vi "MH_CalcDeltaT_EB.vi"(0 "WinDelta":i32, 1 "TrueTime":u64, 2 "WIndowW":i32, 3 "Buffsize":i32, 4 "DBuffSize":i32=10, 5 "Data In":u64[](array[numeric]), 7 "DeltasBuffer":i32[](array[numeric]), 9 "Deltaindex":i32, 11 "error In":errorcluster, 12 "WinIndex":i32, 13 "queue out":refnum<queue>) -> (6 "DeltasBufferOut":i32[](array[numeric]), 8 "DeltaIndexOut":i32, 10 "NewDelta":bool, 14 "WinIndexOut":i32, 15 "Error Out":errorcluster caption="error Out")   [LabVIEW 2019]
uses:
  <userlib>/MultiHarp150/T2Lib/MH_T2DeltaQMessage.ctl
panel:
  # "here"
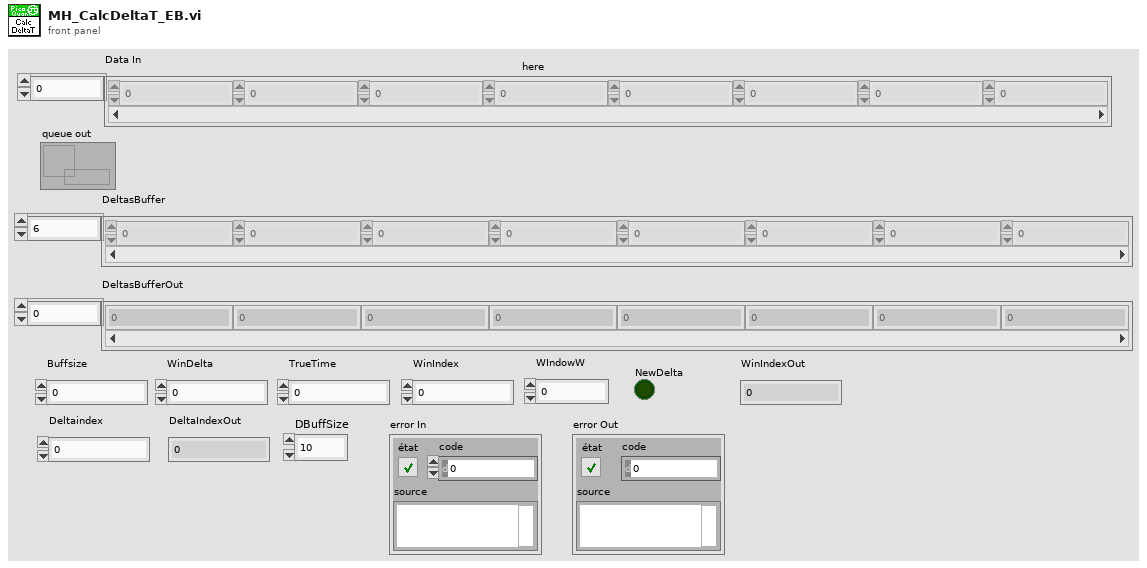
[diagram p1: front panel]
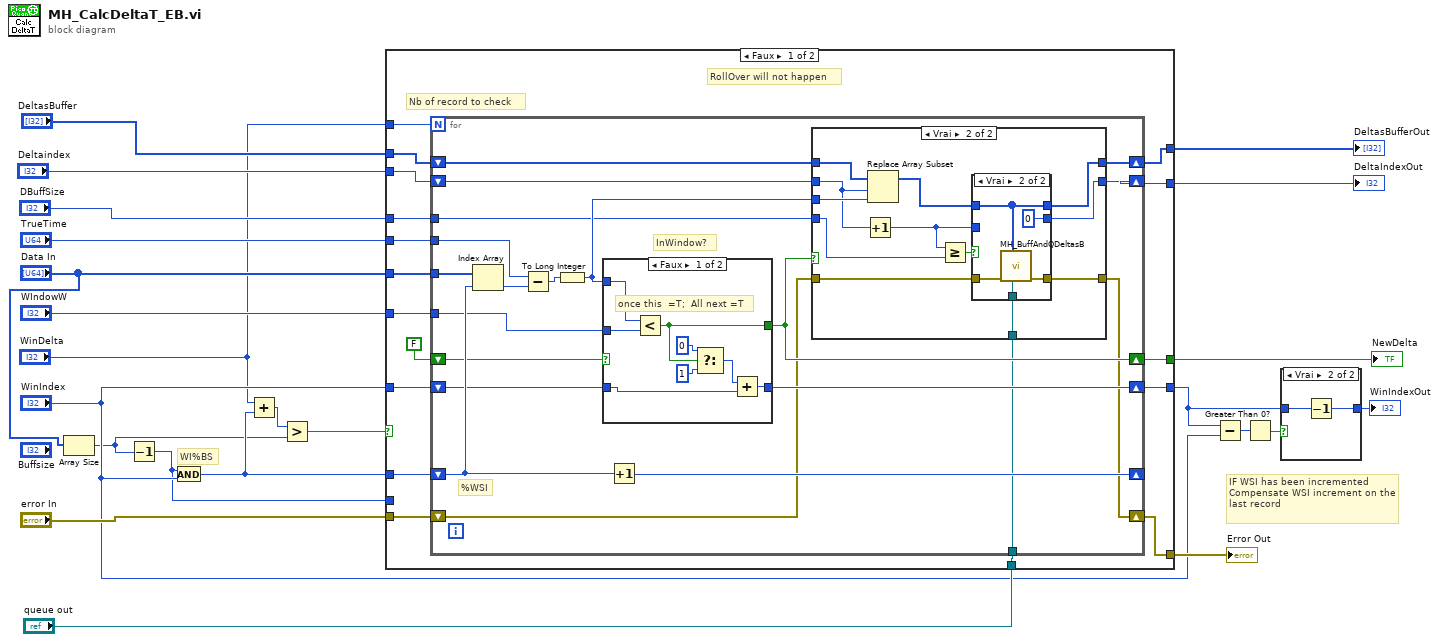
[diagram p0: block diagram]
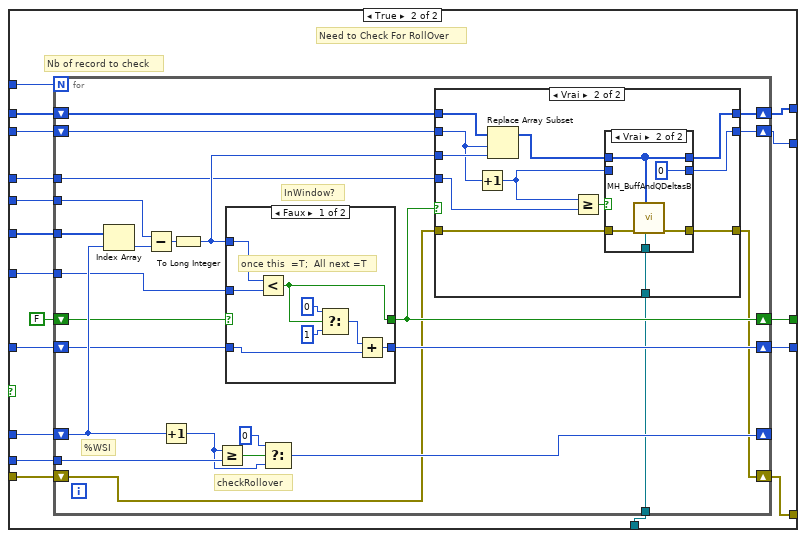
[diagram p5: hidden frame]
diagram:
  # "WI%BS"
  # "IF WSI has been incremented\nCompensate WSI increment on the last record"
  n1 = Array Size(array="Data In") -> (size(s)=w4:i32)
  n2 = Decrement(x=w4) -> (x-1=w5:i32)
  n3 = And(x=w5, y="WinIndex") -> (x .and. y?=w17:i32)
  n4 = Add(x="WinDelta", y=w17) -> (x+y=w16:i32)
  n5 = Greater?(x=w16, y=w4) -> (0:w15:bool)
  n6 = case shown="Faux" w15 {
    tunnel: "Data In" -> [w40 w111]
    tunnel: "TrueTime" -> [w39 w110]
    tunnel: "WIndowW" -> [w38 w109]
    tunnel: [w37 w108] -> w22
    tunnel: "WinIndex" -> [w35 w106]
    tunnel: [w34 w105] -> w18
    tunnel: "WinDelta" -> [w33 w96]
    tunnel: w17 -> [w32 w104]
    tunnel: w5 -> [_ w103]
    tunnel: "DeltasBuffer" -> [w31 w102]
    tunnel: "Deltaindex" -> [w30 w101]
    tunnel: [w28 w100] -> w14
    tunnel: [w29 w99] -> w13
    tunnel: "DBuffSize" -> [w27 w95]
    tunnel: "queue out" -> [w26 w94]
    tunnel: "error In" -> [w25 w98]
    tunnel: [w24 w97] -> w7
    frame False {
      # "RollOver will not happen"
      # "Nb of record to check"
      n7 = for {
        N: w33 -> [_]
        tunnel: w40 -> [w60]
        tunnel: w39 -> [w51]
        shift-right: [w54] -> w34
        shift-left: w35 -> [w55]
        shift-right: [w53] -> _
        shift-left: w32 -> [w58]
        tunnel: w38 -> [w57]
        shift-right: [w45] -> w37
        shift-left: FALSE -> [w56]
        shift-right: [w47] -> w28
        shift-left: w31 -> [w50]
        shift-right: [w46] -> w29
        shift-left: w30 -> [w49]
        tunnel: w27 -> [w44]
        tunnel: w26 -> [w43]
        shift-right: [w42] -> w24
        shift-left: w25 -> [w41]
        # "InWindow?"
        # "%WSI"
        n8 = Index Array(array=w60, index=w58) -> (element=w52:u64)
        n9 = Subtract(x=w51, y=w52) -> (x-y=w59:u64)
        n10 = To Long Integer(number=w59) -> (32bit integer=w48:i32)
        n11 = case shown="Faux" w56 {
          selector: w56 -> [_ w92]
          tunnel: w48 -> [w91 _]
          tunnel: w57 -> [w90 _]
          tunnel: [w86 w92] -> w45
          tunnel: w55 -> [w85 w93]
          tunnel: [w84 w93] -> w54
          frame False {
            # "once this  =T;  All next =T"
            n12 = Less?(x=w91, y=w90) -> (x < y?=w86:bool)
            n13 = Select(t=0 ("WinIndex"), s=w86, f=1 ("WinIndex")) -> (s? t:f=w87:i32)
            n14 = Add(x=w87, y=w85) -> (x+y=w84:i32)
          }
          frame True {
          }
        }
        n15 = Increment(x=w58) -> (x+1=w53:i32)
        n16 = case shown="Vrai" w45 {
          tunnel: w50 -> [w63 w74]
          tunnel: w48 -> [_ w75]
          tunnel: w49 -> [w62 w73]
          tunnel: [w62 w65] -> w46
          tunnel: [w63 w64] -> w47
          tunnel: w44 -> [_ w67]
          tunnel: w43 -> [_ w71]
          tunnel: [w61 w70] -> w42
          tunnel: w41 -> [w61 w69]
          frame False {
          }
          frame True {
            n17 = Increment(x=w73) -> (x+1=w66:i32)
            n18 = Replace Array Subset(array=w74, new element=w75, index=w73) -> (w68:i32[])
            n19 = Greater Or Equal?(x=w66, y=w67) -> (x >= y?=w72:bool)
            n20 = case shown="Vrai" w72 {
              tunnel: w71 -> [_ w83]
              tunnel: [w78 w82] -> w70
              tunnel: w69 -> [w78 w81]
              tunnel: w68 -> [w76 w79]
              tunnel: w66 -> [w77 _]
              tunnel: [w77 0] -> w65
              tunnel: [w76 w79] -> w64
              frame False {
              }
              frame True {
                n21 = call <userlib>:"MH_BuffAndQDeltasB.vi"("queue out"=w83, "DeltasBuffer"=w79, "erroIn"=w81) -> ("error out"=w82:errorcluster)  [unwired: 8 in]
              }
            }
          }
        }
      }
    }
    frame True {
      # "Need to Check For RollOver"
      # "Nb of record to check"
      n22 = for {
        N: w96 -> [_]
        tunnel: w111 -> [w135]
        tunnel: w110 -> [w122]
        shift-right: [w128] -> w105
        shift-left: w106 -> [w129]
        shift-right: [w132] -> _
        shift-left: w104 -> [w133]
        tunnel: w103 -> [w134]
        tunnel: w109 -> [w131]
        shift-right: [w118] -> w108
        shift-left: FALSE -> [w130]
        shift-right: [w121] -> w100
        shift-left: w102 -> [w119]
        shift-right: [w120] -> w99
        shift-left: w101 -> [w117]
        shift-right: [w114] -> w97
        shift-left: w98 -> [w115]
        tunnel: w95 -> [w113]
        tunnel: w94 -> [w112]
        # "InWindow?"
        # "checkRollover"
        # "%WSI"
        n23 = Index Array(array=w135, index=w133) -> (element=w123:u64)
        n24 = Subtract(x=w122, y=w123) -> (x-y=w124:u64)
        n25 = Increment(x=w133) -> (x+1=w125:i32)
        n26 = To Long Integer(number=w124) -> (32bit integer=w116:i32)
        n27 = Greater Or Equal?(x=w125, y=w134) -> (x >= y?=w127:bool)
        n28 = case shown="Faux" w130 {
          selector: w130 -> [_ w167]
          tunnel: w116 -> [w166 _]
          tunnel: w131 -> [w165 _]
          tunnel: [w160 w167] -> w118
          tunnel: w129 -> [w161 w168]
          tunnel: [w159 w168] -> w128
          frame False {
            # "once this  =T;  All next =T"
            n29 = Less?(x=w166, y=w165) -> (x < y?=w160:bool)
            n30 = Select(t=0 ("WinIndex"), s=w160, f=1 ("WinIndex")) -> (s? t:f=w162:i32)
            n31 = Add(x=w162, y=w161) -> (x+y=w159:i32)
          }
          frame True {
          }
        }
        n32 = Select(t=0 ("x+1"), s=w127, f=w125) -> (s? t:f=w132:i32)
        n33 = case shown="Vrai" w118 {
          tunnel: w119 -> [w138 w149]
          tunnel: w116 -> [_ w150]
          tunnel: w117 -> [w137 w148]
          tunnel: [w137 w147] -> w120
          tunnel: [w138 w139] -> w121
          tunnel: w115 -> [w136 w145]
          tunnel: [w136 w144] -> w114
          tunnel: w113 -> [_ w142]
          tunnel: w112 -> [_ w140]
          frame False {
          }
          frame True {
            n34 = Increment(x=w148) -> (x+1=w143:i32)
            n35 = Replace Array Subset(array=w149, new element=w150, index=w148) -> (w141:i32[])
            n36 = Greater Or Equal?(x=w143, y=w142) -> (x >= y?=w146:bool)
            n37 = case shown="Vrai" w146 {
              tunnel: w140 -> [_ w158]
              tunnel: [w153 w157] -> w144
              tunnel: w145 -> [w153 w156]
              tunnel: w141 -> [w151 w154]
              tunnel: w143 -> [w152 _]
              tunnel: [w152 0] -> w147
              tunnel: [w151 w154] -> w139
              frame False {
              }
              frame True {
                n38 = call <userlib>:"MH_BuffAndQDeltasB.vi"("queue out"=w158, "DeltasBuffer"=w154, "erroIn"=w156) -> ("error out"=w157:errorcluster)  [unwired: 8 in]
              }
            }
          }
        }
      }
    }
  }
  "NewDelta" <- w22
  "DeltasBufferOut" <- w14
  "DeltaIndexOut" <- w13
  "Error Out" <- w7
  n39 = Subtract(x=w18, y="WinIndex") -> (x-y=w21:i32)
  n40 = Greater Than 0?(x=w21) -> (x > 0?=w20:bool)
  n41 = case shown="Vrai" w20 {
    tunnel: [w169 w170] -> w19
    tunnel: w18 -> [w169 w171]
    frame False {
    }
    frame True {
      n42 = Decrement(x=w171) -> (x-1=w170:i32)
    }
  }
  "WinIndexOut" <- w19
